vi "Begin.vi"() -> (0 "CameraDevRef 2":T1, 1 "CameraDevRef":T1)   [LabVIEW 2011]
doc: "Called before other user functions, this VI is expected to open initial I/O refnums, load in file data, and do all program initialization. Notice that the <B>error out</B> terminal is simply used for data flow. Wiring it to other structures or subVIs ensures that this VI runs first."
uses:
  <vilib>/Rock Robotics/WPI/Camera/WPI_CameraDevRef.ctl
  <vilib>/Rock Robotics/SystemInterfaces/DIO/FPGA_DIOPWMChannel.ctl
  <vilib>/Rock Robotics/WPI/Joystick/WPI_JoystickDeviceEnum.ctl
  <vilib>/Rock Robotics/SystemInterfaces/AI/FPGA_AIChannel.ctl
  <vilib>/Rock Robotics/SystemInterfaces/DIO/FPGA_DIORelayChannel.ctl
  <vilib>/Rock Robotics/SystemInterfaces/DIO/FPGA_DIOChannel.ctl
  <vilib>/Rock Robotics/SystemInterfaces/AI/FPGA_AIGyroChannel.ctl
  <vilib>/Rock Robotics/WPI/Relay/WPI_RelayDirection.ctl
  <vilib>/Rock Robotics/WPI/Encoder/WPI_EncoderType.ctl
  <vilib>/Rock Robotics/WPI/DriverStation/DriverStationLCD/WPI_DriverStationLCDLCDLine.ctl
  <vilib>/Rock Robotics/WPI/MotorControl/WPI_MotorControlOpen Victor.vi
  <vilib>/Rock Robotics/WPI/MotorControl/WPI_MotorControlOpen Jaguar.vi
  Robot Global Data.vi
  <vilib>/Utility/file.llb/Read From Spreadsheet File (DBL).vi
  <vilib>/Rock Robotics/WPI/Counter/WPI_CounterDigitalInputToDigitalSource.vi
  <vilib>/Rock Robotics/SystemInterfaces/Typedef/FPGA_TypedefDigitalModule.ctl
  <vilib>/Rock Robotics/SystemInterfaces/Typedef/FPGA_TypedefAnalogModule.ctl
panel:
  in  "Default Shooter in Feet":i32=13
  out "Path and file":string
  in  "Balls In Robot At Start":dbl=2.0
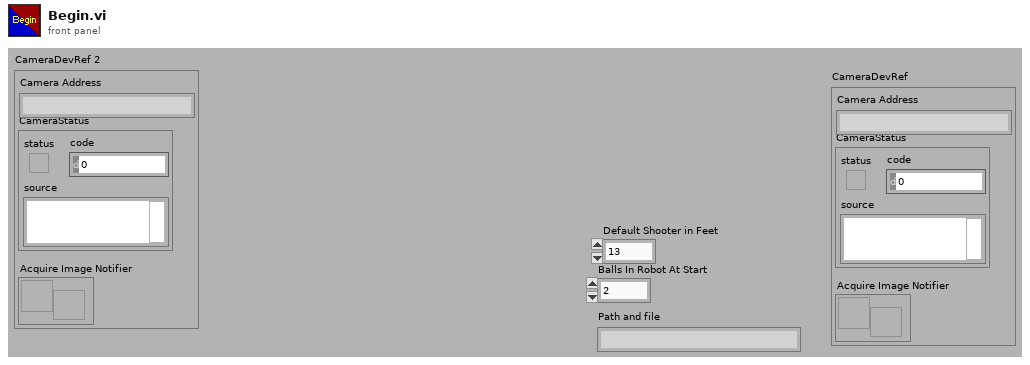
[diagram p1: front panel]
types:
  T1 = typedef "WPI_CameraDevRef.ctl" = cluster{"Camera Address":string, "CameraStatus":errorcluster, "Acquire Image Notifier":refnum<notifier>}
  T2 = typedef "FPGA_DIOPWMChannel.ctl" = enum8{"PWM 1", "PWM 2", "PWM 3", "PWM 4", "PWM 5", "PWM 6", "PWM 7", "PWM 8", "PWM 9", "PWM 10", "Invalid"}
  T3 = typedef "WPI_DriverStationLCDLCDLine.ctl" = enum16{"Main - Line 1", "User - Line 2", "User - Line 3", "User - Line 4", "User - Line 5", "User - Line 6"}
  T4 = typedef "WPI_EncoderType.ctl" = enum16{"1x", "2x", "4x"}
  T5 = typedef "FPGA_DIOChannel.ctl" = enum8{"DIO 1", "DIO 2", "DIO 3", "DIO 4", "DIO 5", "DIO 6", "DIO 7", "DIO 8", "DIO 9", "DIO 10", "DIO 11", "DIO 12", "DIO 13", "DIO 14", "Invalid"}
  T6 = typedef "FPGA_DIORelayChannel.ctl" = enum8{"Relay 1", "Relay 2", "Relay 3", "Relay 4", "Relay 5", "Relay 6", "Relay 7", "Relay 8", "Invalid"}
  T7 = typedef "WPI_RelayDirection.ctl" = enum16{"Both directions", "Forward only", "Reverse only"}
  T8 = typedef "FPGA_AIGyroChannel.ctl" = enum8{"AI 1", "AI 2", "Invalid"}
  T9 = typedef "FPGA_AIChannel.ctl" = enum8{"AI 1", "AI 2", "AI 3", "AI 4", "AI 5", "AI 6", "AI 7", "AI 8", "Invalid"}
  T10 = typedef "WPI_JoystickDeviceEnum.ctl" = enum16{"USB 1", "USB 2", "USB 3", "USB 4", "Kinect 1", "Kinect 2"}
  T11 = typedef "WPI_CameraImageSize.ctl" = enum16{"640x480", "320x240", "160x120"}
  T12 = cluster{"fps":i32, "compression":i32, "Image Size":T11}
  T13 = typedef "WPI_MotorControlDeviceRef.ctl" = cluster{"DeviceStatus":errorcluster, "Type":enum16{"PWM", "CAN"}, "PWM":cluster{"Digital Module":T14, "PWM Channel":T2, "DeadBand":T15}, "CAN":cluster{"Device Number":u8, "Control Mode":T16, "Semaphore":T17, "Max Vout":dbl}, "Invert":bool, "TransformRef":T18, "InvTransformRef":T18}
  T14 = typedef "FPGA_TypedefDigitalModule.ctl" = enum16{"Digital Module 1", "Digital Module 2"}
  T15 = typedef "WPI_PWMDeadband.ctl" = cluster{"Name":string, "maxPositivePwm":i32, "minPositivePwm":i32, "centerPwm":i32, "maxNegativePwm":i32, "minNegativePwm":i32, "angularRange":u16}
  T16 = typedef "WPI_CANJaguar_ControlMode.ctl" = enum8{"Percent VBus", "Current", "Speed", "Position", "Voltage"}
  T17 = typedef "Semaphore RefNum" = refnum<k1>
  T18 = typedef "WPI_PWMTransform_ConPane.ctl" = refnum<vi>
  T19 = typedef "WPI_ServoDeviceRef.ctl" = cluster{"DeviceStatus":errorcluster, "Digital Module":T14, "PWM Channel":T2, "DeadBand":T15}
  T20 = typedef "WPI_AnalogChannelDevRef.ctl" = cluster{"DevStatus":errorcluster, "Analog Module":T21, "Analog Channel":T9}
  T21 = typedef "FPGA_TypedefAnalogModule.ctl" = enum16{"Analog Module 1", "Analog Module 2"}
  T22 = typedef "WPI_CameraWhite Balance Values.ctl" = enum16{"Auto", "Fixed indoor", "Fixed outdoor 1", "Fixed outdoor 2", "Fixed fluorescent 1", "Fixed fluorescent 2", "Hold current"}
  T23 = typedef "WPI_JoystickDevRef.ctl" = cluster{"Device":T10}
  T24 = typedef "WPI_RelayDevRef.ctl" = cluster{"DevStatus":errorcluster, "Relay Channel":T6, "Digital Module":T14, "Relay Direction":T7}
  T25 = typedef "WPI_CameraExposure Values.ctl" = enum16{"Auto", "Flicker-free 50 Hz", "Flicker-free 60 Hz", "Hold current"}
  T26 = typedef "WPI_DigitalInputDevRef.ctl" = cluster{"DevStatus":errorcluster, "DIO Channel":T5, "Digital Module":T14}
  T27 = typedef "FPGA_CounterEncoderSourceConvertionLVSourceType.ctl" = cluster{"DevStatus":errorcluster, "AnalogTriggerMode?":bool, "DigitalMode":cluster{"Digital Module":T14, "DIO Channel":T28}, "AnalogTriggerMode":cluster{"AnalogTriggerIndex":T29, "OutputType":T30}}
  T28 = typedef "FPGA_DIODigitalSourceChannel.ctl" = enum8{"DIO 1", "DIO 2", "DIO 3", "DIO 4", "DIO 5", "DIO 6", "DIO 7", "DIO 8", "DIO 9", "DIO 10", "DIO 11", "DIO 12", "DIO 13", "DIO 14", "Disabled"}
  T29 = typedef "FPGA_AnalogTriggerIndex.ctl" = enum8{"Trig 0", "Trig 1", "Trig 2", "Trig 3", "Trig 4", "Trig 5", "Trig 6", "Trig 7", "Invalid"}
  T30 = typedef "FPGA_AnalogTriggerOutType.ctl" = enum16{"InWindow", "TriggerState", "Rising", "Falling"}
  T31 = typedef "WPI_EncoderDevRef.ctl" = cluster{"DevStatus":errorcluster, "EncoderIndex":T32, "CounterIndex":T33, "DistancePerCount":dbl, "Decoding Type":T4}
  T32 = typedef "FPGA_EncoderIdx.ctl" = enum8{"Enc 0", "Enc 1", "Enc 2", "Enc 3", "Invalid"}
  T33 = typedef "FPGA_CounterCtrSystemIndex.ctl" = enum8{"Ctr 0", "Ctr 1", "Ctr 2", "Ctr 3", "Ctr 4", "Ctr 5", "Ctr 6", "Ctr 7", "Invalid"}
  T34 = typedef "WPI_UltrasonicDeviceRef.ctl" = cluster{"DevStatus":errorcluster, "Ping Digital Module":T14, "Echo Digital Module":T14, "Ping Channel":T5, "Echo Channel":T5, "CntIndex":T33}
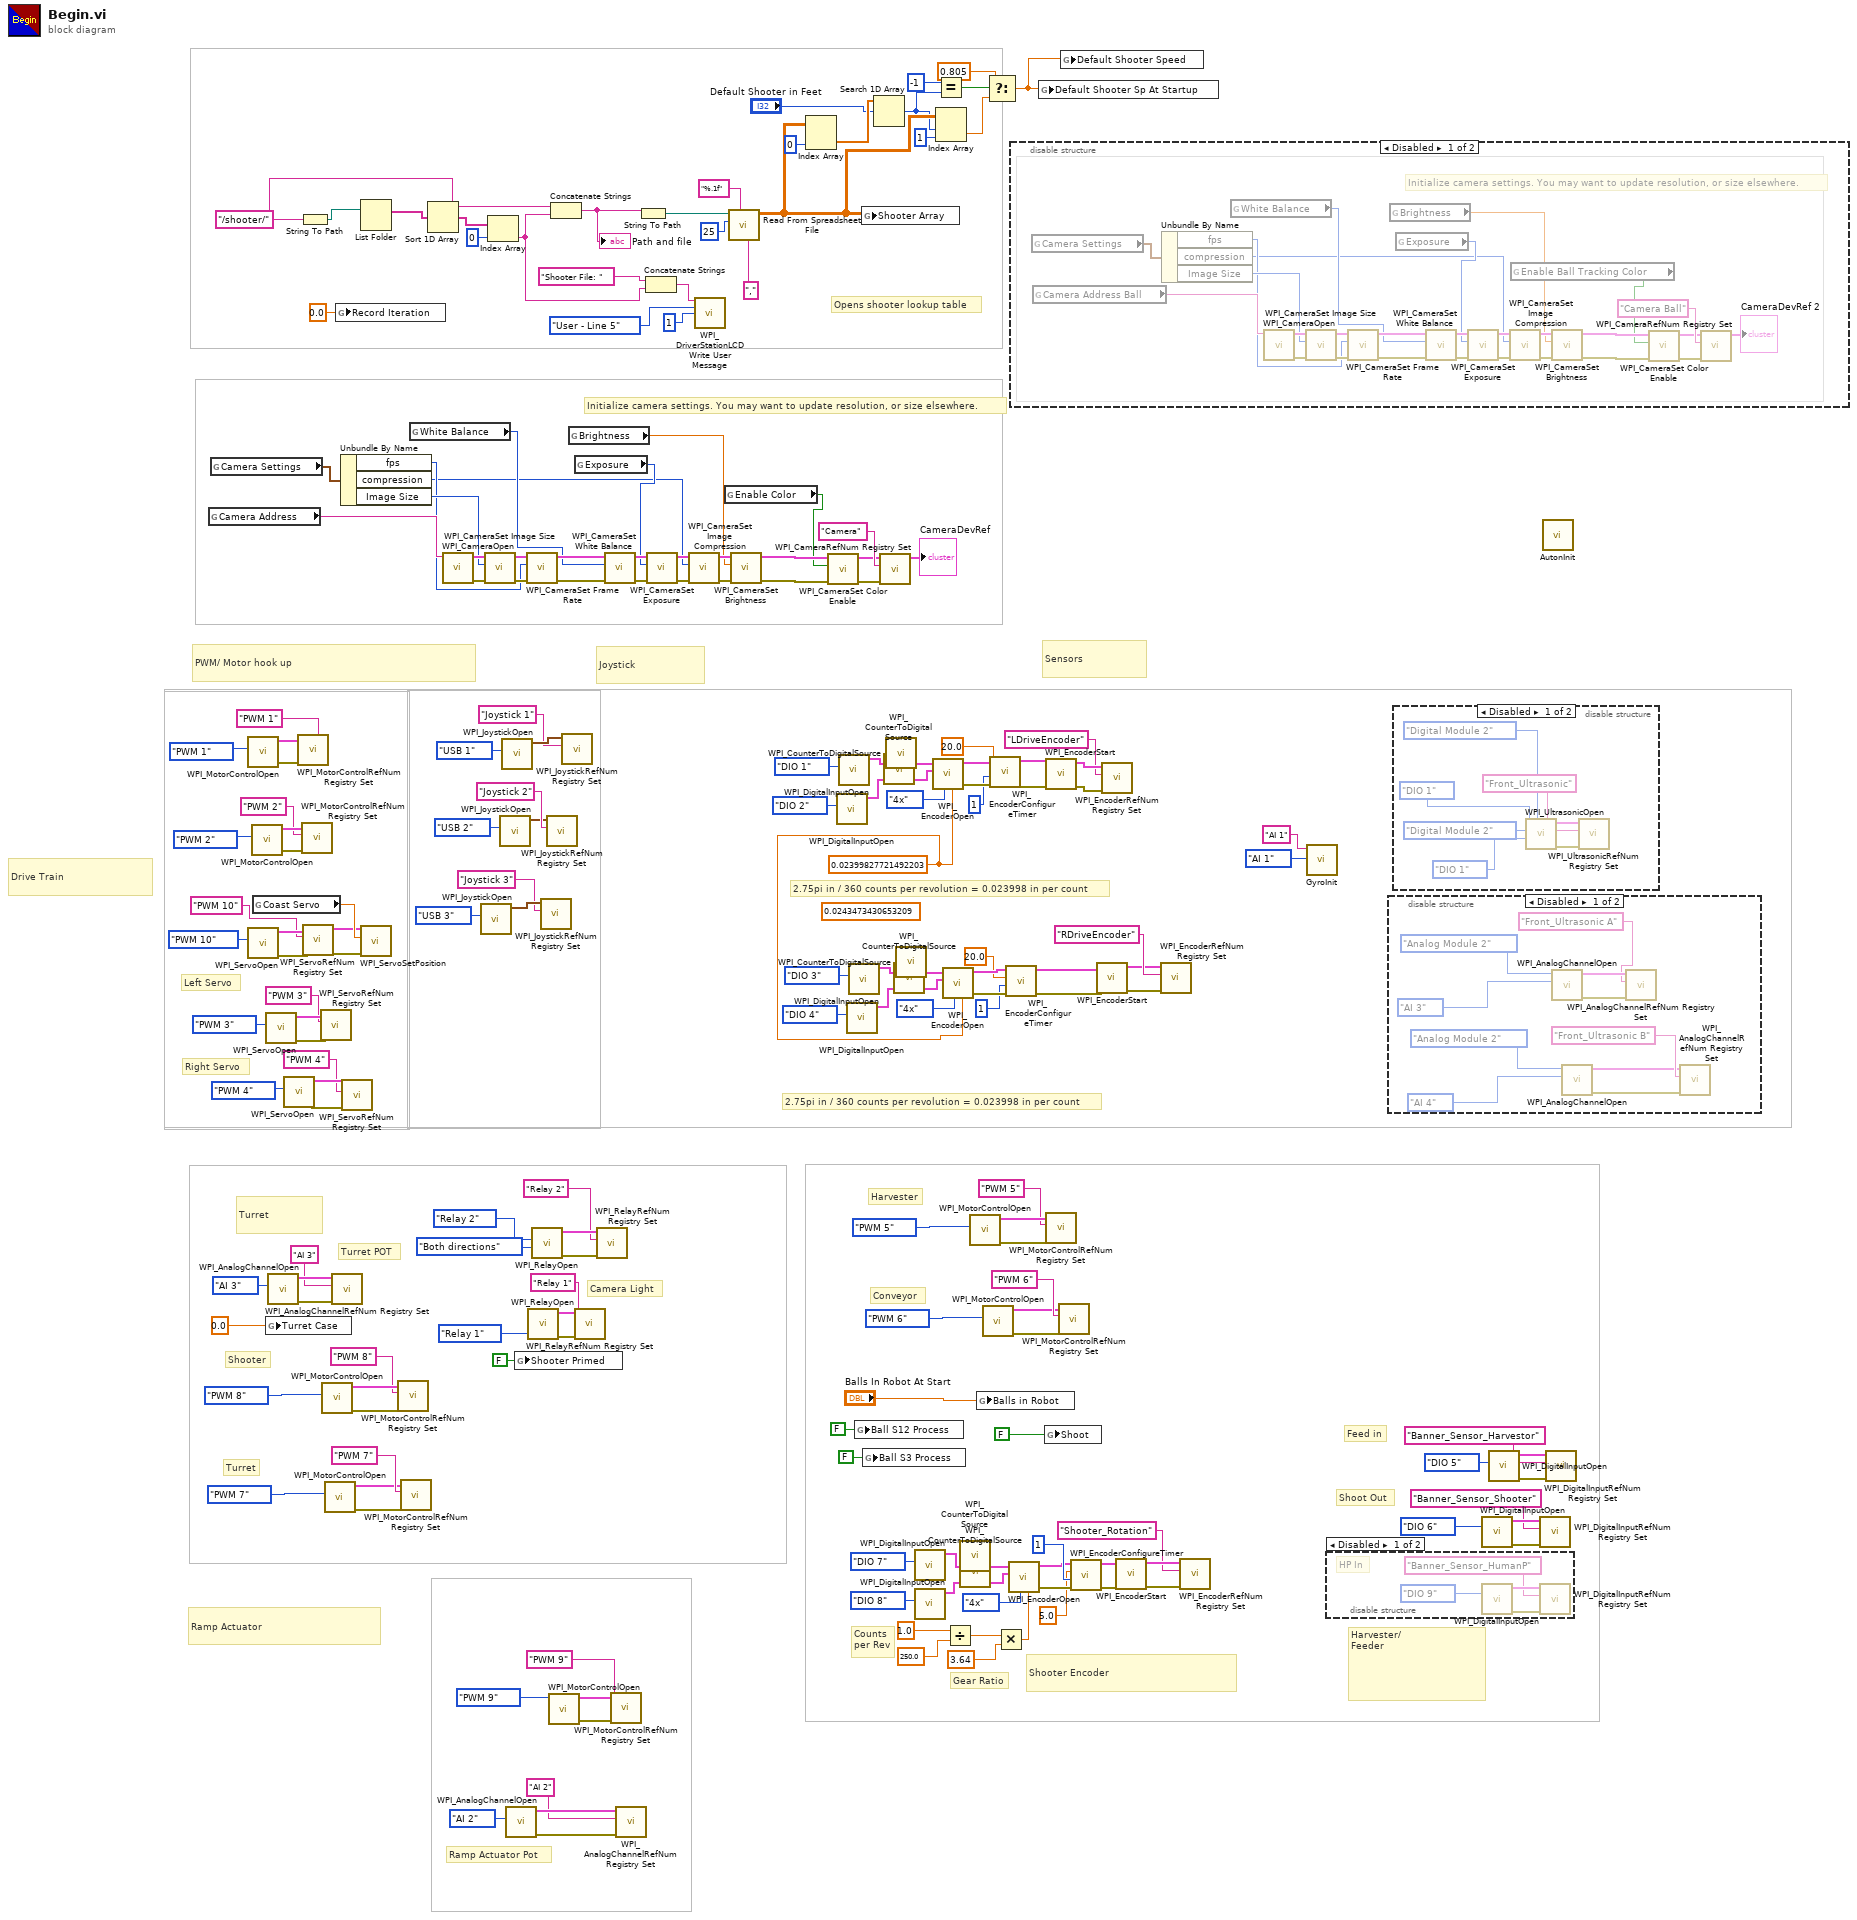
[diagram p0: block diagram]
diagram:
  (unwired) 0.0243473430653209 ("DistancePerCount")
  w45 = 0.02399827721492203 ("DistancePerCount")
  w85 = "/shooter/" ("string")
  # "Shooter Encoder"
  # "Counts\nper Rev"
  # "Gear Ratio"
  # "2.75pi in / 360 counts per revolution = 0.023998 in per count"
  # "2.75pi in / 360 counts per revolution = 0.023998 in per count"
  # "Opens shooter lookup table"
  # "Shoot Out"
  # "Feed in"
  # "Harvester"
  # "Conveyor"
  # "Shooter"
  # "Initialize camera settings. You may want to update resolution, or size elsewhere."
  # "Camera Light"
  # "Ramp Actuator Pot"
  # "Turret POT"
  # "Turret"
  # "Right Servo"
  # "Left Servo"
  # "Harvester/\nFeeder"
  # "Turret"
  # "Ramp Actuator"
  # "Drive Train"
  # "Sensors"
  # "Joystick"
  # "PWM/ Motor hook up"
  n1 = global read "Robot Global Data.vi" "Camera Address"() -> (w134:string)
  n2 = global read "Robot Global Data.vi" "Camera Settings"() -> (w133:T12)
  n3 = call-poly <vilib>:"WPI_MotorControlOpen.vi"("PWM Channel"=FPGA_DIOPWMChannel."PWM 1") -> ("error out"=w174:errorcluster, "MotorControlDeviceRef"=w176:T13)  [unwired: 9 in]
  n4 = call <vilib>:"WPI_ServoOpen.vi"("PWM Channel"=FPGA_DIOPWMChannel."PWM 10") -> ("error out"=w13:errorcluster, "ServoDeviceRef"=w17:T19)  [unwired: 9 in]
  n5 = call-poly <vilib>:"WPI_MotorControlOpen.vi"("PWM Channel"=FPGA_DIOPWMChannel."PWM 2") -> ("error out"=w172:errorcluster, "MotorControlDeviceRef"=w170:T13)  [unwired: 9 in]
  n6 = global read "Robot Global Data.vi" "Coast Servo"() -> (w18:dbl)
  n7 = call <vilib>:"WPI_ServoOpen.vi"("PWM Channel"=FPGA_DIOPWMChannel."PWM 3") -> ("error out"=w187:errorcluster, "ServoDeviceRef"=w192:T19)  [unwired: 9 in]
  n8 = global write "Robot Global Data.vi" "Turret Case"(0.0 ("Return To Home Case")) -> ()
  n9 = call <vilib>:"WPI_AnalogChannelOpen.vi"("Analog Channel"=FPGA_AIChannel."AI 3") -> ("error out"=w163:errorcluster, "AIDeviceRef"=w164:T20)  [unwired: 9 in]
  n10 = call <vilib>:"WPI_ServoOpen.vi"("PWM Channel"=FPGA_DIOPWMChannel."PWM 4") -> ("error out"=w186:errorcluster, "ServoDeviceRef"=w190:T19)  [unwired: 9 in]
  n11 = call <vilib>:"WPI_MotorControlRefNum Registry Set.vi"("error in (no error)"=w174, "refnum name"="PWM 1", "MotorControlDevRef"=w176) -> ()  [unwired: 7 in, 2 out]
  n12 = String To Path(string=w85) -> (path=w94:path)
  n13 = call <vilib>:"WPI_MotorControlRefNum Registry Set.vi"("error in (no error)"=w172, "refnum name"="PWM 2", "MotorControlDevRef"=w170) -> ()  [unwired: 7 in, 2 out]
  n14 = call <vilib>:"WPI_ServoRefNum Registry Set.vi"("error in (no error)"=w13, "refnum name"="PWM 10", "ServoDeviceRef"=w17) -> ("error out"=w14:errorcluster, "ServoDeviceRef"=w15:T19)  [unwired: 7 in]
  n15 = call <vilib>:"WPI_ServoRefNum Registry Set.vi"("error in (no error)"=w187, "refnum name"="PWM 3", "ServoDeviceRef"=w192) -> ()  [unwired: 7 in, 2 out]
  n16 = call-poly <vilib>:"WPI_MotorControlOpen.vi"("PWM Channel"=FPGA_DIOPWMChannel."PWM 8") -> ("error out"=w117:errorcluster, "MotorControlDeviceRef"=w119:T13)  [unwired: 9 in]
  n17 = call-poly <vilib>:"WPI_MotorControlOpen.vi"("PWM Channel"=FPGA_DIOPWMChannel."PWM 7") -> ("error out"=w168:errorcluster, "MotorControlDeviceRef"=w166:T13)  [unwired: 9 in]
  n18 = call <vilib>:"WPI_AnalogChannelRefNum Registry Set.vi"("error in (no error)"=w163, "refnum name"="AI 3", "AIDeviceRef"=w164) -> ()  [unwired: 7 in, 2 out]
  n19 = global write "Robot Global Data.vi" "Record Iteration"(0.0 ("Record Iteration")) -> ()
  n20 = Unbundle By Name(w133) -> ("fps"=w131:i32, "compression"=w128:i32, "Image Size"=w132:T11)
  n21 = call <vilib>:"WPI_ServoRefNum Registry Set.vi"("error in (no error)"=w186, "refnum name"="PWM 4", "ServoDeviceRef"=w190) -> ()  [unwired: 7 in, 2 out]
  n22 = List Folder(path=w94) -> (filenames=w93:string[])  [unwired: 1 in, 5 out]
  n23 = call <vilib>:"WPI_ServoSetPosition.vi"("error in (no error)"=w14, "Position"=w18, "ServoDeviceRef"=w15) -> ()  [unwired: 7 in, 2 out]
  n24 = call <vilib>:"WPI_MotorControlRefNum Registry Set.vi"("error in (no error)"=w117, "refnum name"="PWM 8", "MotorControlDevRef"=w119) -> ()  [unwired: 7 in, 2 out]
  n25 = call <vilib>:"WPI_MotorControlRefNum Registry Set.vi"("error in (no error)"=w168, "refnum name"="PWM 7", "MotorControlDevRef"=w166) -> ()  [unwired: 7 in, 2 out]
  n26 = global read "Robot Global Data.vi" "White Balance"() -> (w130:T22)
  n27 = Sort 1D Array(array=w93) -> (sorted array=w92:string[])
  n28 = call <vilib>:"WPI_CameraOpen.vi"("Camera Address"=w134) -> ("error out"=w140:errorcluster, "CameraDevRef"=w141:T1)  [unwired: 1 in, 8 out]
  n29 = call <vilib>:"WPI_JoystickOpen.vi"("JoystickDevice"=WPI_JoystickDeviceEnum."USB 3") -> ("JoystickDevRef"=w179:T23)  [unwired: 10 in]
  n30 = call <vilib>:"WPI_CameraSet Image Size.vi"("error in (no error)"=w140, "Image Size"=w132, "CameraDevRef"=w141) -> ("error out"=w139:errorcluster, "CameraDevRef Out"=w142:T1)  [unwired: 7 out]
  n31 = Index Array(array=w92, index=0) -> (element=w21:string)
  n32 = call <vilib>:"WPI_JoystickOpen.vi"("JoystickDevice"=WPI_JoystickDeviceEnum."USB 2") -> ("JoystickDevRef"=w182:T23)  [unwired: 10 in]
  n33 = call <vilib>:"WPI_JoystickOpen.vi"("JoystickDevice"=WPI_JoystickDeviceEnum."USB 1") -> ("JoystickDevRef"=w185:T23)  [unwired: 10 in]
  n34 = call <vilib>:"WPI_AnalogChannelOpen.vi"("Analog Channel"=FPGA_AIChannel."AI 2") -> ("error out"=w158:errorcluster, "AIDeviceRef"=w159:T20)  [unwired: 9 in]
  n35 = global write "Robot Global Data.vi" "Shooter Primed"(FALSE ("Ball S3 Process")) -> ()
  n36 = call <vilib>:"WPI_CameraSet Frame Rate.vi"("error in (no error)"=w139, "Frame Rate (fps)"=w131, "CameraDevRef"=w142) -> ("error out"=w138:errorcluster, "CameraDevRef Out"=w144:T1)  [unwired: 7 out]
  n37 = call <vilib>:"WPI_RelayOpen.vi"("Relay Channel"=FPGA_DIORelayChannel."Relay 1") -> ("error out"=w151:errorcluster, "RelayDevRef"=w150:T24)  [unwired: 9 in]
  n38 = call <vilib>:"WPI_RelayOpen.vi"("Relay Direction"=WPI_RelayDirection."Both directions", "Relay Channel"=FPGA_DIORelayChannel."Relay 2") -> ("error out"=w81:errorcluster, "RelayDevRef"=w82:T24)  [unwired: 8 in]
  n39 = call <vilib>:"WPI_JoystickRefNum Registry Set.vi"("refnum name"="Joystick 3", "JoystickDevRef"=w179) -> ()  [unwired: 8 in, 2 out]
  n40 = call <vilib>:"WPI_JoystickRefNum Registry Set.vi"("refnum name"="Joystick 2", "JoystickDevRef"=w182) -> ()  [unwired: 8 in, 2 out]
  n41 = call-poly <vilib>:"WPI_MotorControlOpen.vi"("PWM Channel"=FPGA_DIOPWMChannel."PWM 9") -> ("error out"=w154:errorcluster, "MotorControlDeviceRef"=w155:T13)  [unwired: 9 in]
  n42 = Concatenate Strings(w85, w21) -> (w87:string)
  "Path and file" <- w87
  n43 = call <vilib>:"WPI_JoystickRefNum Registry Set.vi"("refnum name"="Joystick 1", "JoystickDevRef"=w185) -> ()  [unwired: 8 in, 2 out]
  n44 = global read "Robot Global Data.vi" "Brightness"() -> (w127:dbl)
  n45 = global read "Robot Global Data.vi" "Exposure"() -> (w129:T25)
  n46 = call <vilib>:"WPI_RelayRefNum Registry Set.vi"("error in (no error)"=w151, "refnum name"="Relay 1", "RelayDevRef"=w150) -> ()  [unwired: 7 in, 2 out]
  n47 = call <vilib>:"WPI_RelayRefNum Registry Set.vi"("error in (no error)"=w81, "refnum name"="Relay 2", "RelayDevRef"=w82) -> ()  [unwired: 7 in, 2 out]
  n48 = call <vilib>:"WPI_CameraSet White Balance.vi"("error in (no error)"=w138, "White Balance"=w130, "CameraDevRef"=w144) -> ("error out"=w137:errorcluster, "CameraDevRef Out"=w143:T1)  [unwired: 7 out]
  n49 = call <vilib>:"WPI_MotorControlRefNum Registry Set.vi"("error in (no error)"=w154, "refnum name"="PWM 9", "MotorControlDevRef"=w155) -> ()  [unwired: 7 in, 2 out]
  n50 = call <vilib>:"WPI_AnalogChannelRefNum Registry Set.vi"("error in (no error)"=w158, "refnum name"="AI 2", "AIDeviceRef"=w159) -> ()  [unwired: 7 in, 2 out]
  n51 = String To Path(string=w87) -> (path=w86:path)
  n52 = Concatenate Strings("Shooter File: ", w21) -> (w19:string)
  n53 = call <vilib>:"WPI_CameraSet Exposure.vi"("error in (no error)"=w137, "Exposure"=w129, "CameraDevRef"=w143) -> ("error out"=w136:errorcluster, "CameraDevRef Out"=w146:T1)  [unwired: 7 out]
  n54 = call <vilib>:"WPI_CameraSet Image Compression.vi"("error in (no error)"=w136, "Compression"=w128, "CameraDevRef"=w146) -> ("error out"=w135:errorcluster, "CameraDevRef Out"=w145:T1)  [unwired: 7 out]
  n55 = call <vilib>:"WPI_DriverStationLCDWrite User Message.vi"("line text"=w19, "line"=WPI_DriverStationLCDLCDLine."User - Line 5", "starting column"=i8 1) -> ()  [unwired: 2 in, 11 out]
  n56 = global read "Robot Global Data.vi" "Enable Color"() -> (w122:bool)
  n57 = call-poly <vilib>:"Read From Spreadsheet File.vi"("delimiter (\\t)"="," ("delimiter (\\t)"), "format (%.3f)"="%.1f", "number of rows (all:-1)"=25, "file path (dialog if empty)"=w86) -> ("all rows"=w8:dbl[][])  [unwired: 1 in, 6 out]
  n58 = call <vilib>:"WPI_CameraSet Brightness.vi"("error in (no error)"=w135, "Brightness"=w127, "CameraDevRef"=w145) -> ("error out"=w125:errorcluster, "CameraDevRef Out"=w126:T1)  [unwired: 7 out]
  n59 = Index Array(array=w8, index (col)=0 ("disabled index (col)")) -> (element=w10:dbl[])  [unwired: 1 in]
  n60 = call <vilib>:"WPI_CameraSet Color Enable.vi"("error in (no error)"=w125, "Color Enabled"=w122, "CameraDevRef"=w126) -> ("error out"=w123:errorcluster, "CameraDevRef Out"=w124:T1)  [unwired: 7 in]
  n61 = call <vilib>:"WPI_DigitalInputOpen.vi"("DIO Channel"=FPGA_DIOChannel."DIO 2") -> ("DigitalInputDevRef"=w73:T26)  [unwired: 9 in, 1 out]
  n62 = call <vilib>:"WPI_DigitalInputOpen.vi"("DIO Channel"=FPGA_DIOChannel."DIO 1") -> ("DigitalInputDevRef"=w70:T26)  [unwired: 9 in, 1 out]
  n63 = call <vilib>:"WPI_DigitalInputOpen.vi"("DIO Channel"=FPGA_DIOChannel."DIO 4") -> ("DigitalInputDevRef"=w64:T26)  [unwired: 9 in, 1 out]
  n64 = call <vilib>:"WPI_DigitalInputOpen.vi"("DIO Channel"=FPGA_DIOChannel."DIO 3") -> ("DigitalInputDevRef"=w67:T26)  [unwired: 9 in, 1 out]
  n65 = global write "Robot Global Data.vi" "Ball S12 Process"(FALSE ("Ball S12 Process")) -> ()
  n66 = global write "Robot Global Data.vi" "Shooter Array"(w8) -> ()
  n67 = global write "Robot Global Data.vi" "Ball S3 Process"(FALSE ("Ball S3 Process")) -> ()
  n68 = Search 1D Array(1D array=w10, element="Default Shooter in Feet") -> (index of element=w7:i32)  [unwired: 1 in]
  n69 = call <vilib>:"WPI_CameraRefNum Registry Set.vi"("error in (no error)"=w123, "refnum name"="Camera", "CameraDevRef"=w124) -> ("CameraDevRef"=→"CameraDevRef":T1)  [unwired: 8 out]
  n70 = call-poly <vilib>:"WPI_CounterToDigitalSource.vi"("DigitalInputDevRef"=w73) -> ("Digital Source"=w74:T27)  [unwired: 6 in]
  n71 = call-poly <vilib>:"WPI_CounterToDigitalSource.vi"("DigitalInputDevRef"=w70) -> ("Digital Source"=w69:T27)  [unwired: 6 in]
  n72 = call-poly <vilib>:"WPI_CounterToDigitalSource.vi"("DigitalInputDevRef"=w64) -> ("Digital Source"=w63:T27)  [unwired: 6 in]
  n73 = call-poly <vilib>:"WPI_CounterToDigitalSource.vi"("DigitalInputDevRef"=w67) -> ("Digital Source"=w68:T27)  [unwired: 6 in]
  n74 = call <vilib>:"WPI_DigitalInputOpen.vi"("DIO Channel"=FPGA_DIOChannel."DIO 7") -> ("DigitalInputDevRef"=w29:T26)  [unwired: 9 in, 1 out]
  n75 = call <vilib>:"WPI_DigitalInputOpen.vi"("DIO Channel"=FPGA_DIOChannel."DIO 8") -> ("DigitalInputDevRef"=w32:T26)  [unwired: 9 in, 1 out]
  n76 = call <vilib>:"WPI_EncoderOpen.vi"("DistancePerCount"=w45, "Decoding Type"=WPI_EncoderType."4x", "BSource"=w74, "ASource"=w69) -> ("error out"=w49:errorcluster, "EncoderDevRef"=w52:T31)  [unwired: 6 in]
  n77 = Equal?(x=-1, y=w7) -> (x = y?=w5:bool)
  n78 = Index Array(array=w8, index (row)=w7, index (col)=1) -> (element=w3:dbl)
  n79 = call <vilib>:"WPI_EncoderOpen.vi"("DistancePerCount"=w45, "Decoding Type"=WPI_EncoderType."4x", "BSource"=w63, "ASource"=w68) -> ("error out"=w60:errorcluster, "EncoderDevRef"=w59:T31)  [unwired: 6 in]
  n80 = Divide(x=1.0, y=250.0) -> (x/y=w26:dbl)
  n81 = call-poly <vilib>:"WPI_CounterToDigitalSource.vi"("DigitalInputDevRef"=w29) -> ("Digital Source"=w28:T27)  [unwired: 6 in]
  n82 = call-poly <vilib>:"WPI_CounterToDigitalSource.vi"("DigitalInputDevRef"=w32) -> ("Digital Source"=w33:T27)  [unwired: 6 in]
  n83 = call-poly <vilib>:"WPI_MotorControlOpen.vi"("PWM Channel"=FPGA_DIOPWMChannel."PWM 5") -> ("error out"=w113:errorcluster, "MotorControlDeviceRef"=w115:T13)  [unwired: 9 in]
  n84 = global write "Robot Global Data.vi" "Balls in Robot"("Balls In Robot At Start") -> ()
  n85 = call-poly <vilib>:"WPI_MotorControlOpen.vi"("PWM Channel"=FPGA_DIOPWMChannel."PWM 6") -> ("error out"=w112:errorcluster, "MotorControlDeviceRef"=w110:T13)  [unwired: 9 in]
  n86 = Select(t=0.805, s=w5, f=w3) -> (s? t:f=w1:dbl)
  n87 = call <vilib>:"WPI_EncoderConfigureTimer.vi"("error in (no error)"=w49, "Number Samples to Average"=u8 1, "Minimum Rate"=20.0, "EncoderDevRef"=w52) -> ("error out"=w50:errorcluster, "EncoderDevRef"=w51:T31)  [unwired: 6 in]
  n88 = Multiply(x=w26, y=3.64) -> (x*y=w24:dbl)
  n89 = call <vilib>:"WPI_EncoderConfigureTimer.vi"("error in (no error)"=w60, "Number Samples to Average"=u8 1, "Minimum Rate"=20.0, "EncoderDevRef"=w59) -> ("error out"=w56:errorcluster, "EncoderDevRef"=w57:T31)  [unwired: 6 in]
  n90 = call <vilib>:"WPI_EncoderOpen.vi"("DistancePerCount"=w24, "Decoding Type"=WPI_EncoderType."4x", "BSource"=w33, "ASource"=w28) -> ("error out"=w36:errorcluster, "EncoderDevRef"=w37:T31)  [unwired: 6 in]
  n91 = disable-structure shown="Disabled" {
    frame Disabled {
      # "Initialize camera settings. You may want to update resolution, or size elsewhere."
      n92 = global read "Robot Global Data.vi" "Camera Settings"() -> (w206:T12)
      n93 = global read "Robot Global Data.vi" "Camera Address Ball"() -> (w207:string)
      n94 = Unbundle By Name(w206) -> ("fps"=w204:i32, "compression"=w201:i32, "Image Size"=w205:T11)
      n95 = global read "Robot Global Data.vi" "White Balance"() -> (w203:T22)
      n96 = call <vilib>:"WPI_CameraOpen.vi"("Camera Address"=w207) -> ("error out"=w213:errorcluster, "CameraDevRef"=w214:T1)  [unwired: 1 in, 8 out]
      n97 = call <vilib>:"WPI_CameraSet Image Size.vi"("error in (no error)"=w213, "Image Size"=w205, "CameraDevRef"=w214) -> ("error out"=w212:errorcluster, "CameraDevRef Out"=w215:T1)  [unwired: 7 out]
      n98 = call <vilib>:"WPI_CameraSet Frame Rate.vi"("error in (no error)"=w212, "Frame Rate (fps)"=w204, "CameraDevRef"=w215) -> ("error out"=w211:errorcluster, "CameraDevRef Out"=w217:T1)  [unwired: 7 out]
      n99 = global read "Robot Global Data.vi" "Brightness"() -> (w200:dbl)
      n100 = global read "Robot Global Data.vi" "Exposure"() -> (w202:T25)
      n101 = call <vilib>:"WPI_CameraSet White Balance.vi"("error in (no error)"=w211, "White Balance"=w203, "CameraDevRef"=w217) -> ("error out"=w210:errorcluster, "CameraDevRef Out"=w216:T1)  [unwired: 7 out]
      n102 = call <vilib>:"WPI_CameraSet Exposure.vi"("error in (no error)"=w210, "Exposure"=w202, "CameraDevRef"=w216) -> ("error out"=w209:errorcluster, "CameraDevRef Out"=w219:T1)  [unwired: 7 out]
      n103 = call <vilib>:"WPI_CameraSet Image Compression.vi"("error in (no error)"=w209, "Compression"=w201, "CameraDevRef"=w219) -> ("error out"=w208:errorcluster, "CameraDevRef Out"=w218:T1)  [unwired: 7 out]
      n104 = global read "Robot Global Data.vi" "Enable Ball Tracking Color"() -> (w195:bool)
      n105 = call <vilib>:"WPI_CameraSet Brightness.vi"("error in (no error)"=w208, "Brightness"=w200, "CameraDevRef"=w218) -> ("error out"=w198:errorcluster, "CameraDevRef Out"=w199:T1)  [unwired: 7 out]
      n106 = call <vilib>:"WPI_CameraSet Color Enable.vi"("error in (no error)"=w198, "Color Enabled"=w195, "CameraDevRef"=w199) -> ("error out"=w196:errorcluster, "CameraDevRef Out"=w197:T1)  [unwired: 7 in]
      n107 = call <vilib>:"WPI_CameraRefNum Registry Set.vi"("error in (no error)"=w196, "refnum name"="Camera Ball", "CameraDevRef"=w197) -> ("CameraDevRef"=→"CameraDevRef 2":T1)  [unwired: 8 out]
    }
    frame Enabled {
    }
  }
  n108 = global write "Robot Global Data.vi" "Default Shooter Sp At Startup"(w1) -> ()
  n109 = global write "Robot Global Data.vi" "Shoot"(FALSE ("Ball S12 Process")) -> ()
  n110 = call <vilib>:"WPI_EncoderStart.vi"("error in (no error)"=w50, "EncoderDevRef"=w51) -> ("error out"=w77:errorcluster, "EncoderDevRef"=w76:T31)  [unwired: 8 in]
  n111 = call <vilib>:"WPI_MotorControlRefNum Registry Set.vi"("error in (no error)"=w113, "refnum name"="PWM 5", "MotorControlDevRef"=w115) -> ()  [unwired: 7 in, 2 out]
  n112 = call <vilib>:"WPI_MotorControlRefNum Registry Set.vi"("error in (no error)"=w112, "refnum name"="PWM 6", "MotorControlDevRef"=w110) -> ()  [unwired: 7 in, 2 out]
  n113 = global write "Robot Global Data.vi" "Default Shooter Speed"(w1) -> ()
  n114 = call <vilib>:"WPI_EncoderConfigureTimer.vi"("error in (no error)"=w36, "Number Samples to Average"=u8 1, "Minimum Rate"=5.0, "EncoderDevRef"=w37) -> ("error out"=w40:errorcluster, "EncoderDevRef"=w39:T31)  [unwired: 6 in]
  n115 = call <vilib>:"WPI_EncoderStart.vi"("error in (no error)"=w56, "EncoderDevRef"=w57) -> ("error out"=w54:errorcluster, "EncoderDevRef"=w55:T31)  [unwired: 8 in]
  n116 = call <vilib>:"WPI_EncoderRefNum Registry Set.vi"("error in (no error)"=w77, "refnum name"="LDriveEncoder", "EncoderDevRef"=w76) -> ()  [unwired: 7 in, 2 out]
  n117 = call <vilib>:"WPI_EncoderStart.vi"("error in (no error)"=w40, "EncoderDevRef"=w39) -> ("error out"=w42:errorcluster, "EncoderDevRef"=w41:T31)  [unwired: 8 in]
  n118 = call <vilib>:"WPI_EncoderRefNum Registry Set.vi"("error in (no error)"=w54, "refnum name"="RDriveEncoder", "EncoderDevRef"=w55) -> ()  [unwired: 7 in, 2 out]
  n119 = call <vilib>:"WPI_EncoderRefNum Registry Set.vi"("error in (no error)"=w42, "refnum name"="Shooter_Rotation", "EncoderDevRef"=w41) -> ()  [unwired: 7 in, 2 out]
  n120 = call "GyroInit.vi"("refnum name"="AI 1", "Analog Channel"=FPGA_AIGyroChannel."AI 1") -> ()  [unwired: 8 in]
  n121 = disable-structure shown="Disabled" {
    frame Disabled {
      # "HP In"
      n122 = call <vilib>:"WPI_DigitalInputOpen.vi"("DIO Channel"=FPGA_DIOChannel."DIO 9") -> ("error out"=w223:errorcluster, "DigitalInputDevRef"=w222:T26)  [unwired: 9 in]
      n123 = call <vilib>:"WPI_DigitalInputRefNum Registry Set.vi"("error in (no error)"=w223, "refnum name"="Banner_Sensor_HumanP", "DigitalInputDevRef"=w222) -> ()  [unwired: 7 in, 2 out]
    }
    frame Enabled {
    }
  }
  n124 = disable-structure shown="Disabled" {
    frame Disabled {
      n125 = call <vilib>:"WPI_AnalogChannelOpen.vi"("Analog Channel"=FPGA_AIChannel."AI 3", "Analog Module (Module 1)"=FPGA_TypedefAnalogModule."Analog Module 2") -> ("error out"=w230:errorcluster, "AIDeviceRef"=w229:T20)  [unwired: 8 in]
      n126 = call <vilib>:"WPI_AnalogChannelOpen.vi"("Analog Channel"=FPGA_AIChannel."AI 4", "Analog Module (Module 1)"=FPGA_TypedefAnalogModule."Analog Module 2") -> ("error out"=w225:errorcluster, "AIDeviceRef"=w226:T20)  [unwired: 8 in]
      n127 = call <vilib>:"WPI_AnalogChannelRefNum Registry Set.vi"("error in (no error)"=w230, "refnum name"="Front_Ultrasonic A", "AIDeviceRef"=w229) -> ()  [unwired: 7 in, 2 out]
      n128 = call <vilib>:"WPI_AnalogChannelRefNum Registry Set.vi"("error in (no error)"=w225, "refnum name"="Front_Ultrasonic B", "AIDeviceRef"=w226) -> ()  [unwired: 7 in, 2 out]
    }
    frame Enabled {
    }
  }
  n129 = disable-structure shown="Disabled" {
    frame Disabled {
      n130 = call <vilib>:"WPI_UltrasonicOpen.vi"("Ping Digital Module (Module 1)"=FPGA_TypedefDigitalModule."Digital Module 2", "Echo DIO Channel"=FPGA_DIOChannel."DIO 1", "Echo Digital Module (Module 1)"=FPGA_TypedefDigitalModule."Digital Module 2", "Ping DIO Channel"=FPGA_DIOChannel."DIO 1") -> ("error out"=w241:errorcluster, "UltrasonicDevRef"=w240:T34)  [unwired: 6 in]
      n131 = call <vilib>:"WPI_UltrasonicRefNum Registry Set.vi"("error in (no error)"=w241, "refnum name"="Front_Ultrasonic", "UltrasonicDevRef"=w240) -> ()  [unwired: 7 in, 2 out]
    }
    frame Enabled {
    }
  }
  n132 = call <vilib>:"WPI_DigitalInputOpen.vi"("DIO Channel"=FPGA_DIOChannel."DIO 6") -> ("error out"=w103:errorcluster, "DigitalInputDevRef"=w102:T26)  [unwired: 9 in]
  n133 = call <vilib>:"WPI_DigitalInputOpen.vi"("DIO Channel"=FPGA_DIOChannel."DIO 5") -> ("error out"=w106:errorcluster, "DigitalInputDevRef"=w105:T26)  [unwired: 9 in]
  n134 = call <vilib>:"WPI_DigitalInputRefNum Registry Set.vi"("error in (no error)"=w103, "refnum name"="Banner_Sensor_Shooter", "DigitalInputDevRef"=w102) -> ()  [unwired: 7 in, 2 out]
  n135 = call "AutonInit.vi"() -> ()  [unwired: 8 in, 4 out]
  n136 = call <vilib>:"WPI_DigitalInputRefNum Registry Set.vi"("error in (no error)"=w106, "refnum name"="Banner_Sensor_Harvestor", "DigitalInputDevRef"=w105) -> ()  [unwired: 7 in, 2 out]
